vi "Open.vi"(8 "error in (no error)":errorcluster caption="entrée d'erreur (pas d'erreur)", 11 "Class Power_Supply Rigol DP800 en entrée":refnum<class "Class Power_Supply Rigol DP800.lvclass">) -> (0 "error out":errorcluster caption="sortie d'erreur", 3 "Class Power_Supply Rigol DP800 en sortie":refnum<class "Class Power_Supply Rigol DP800.lvclass">)   [LabVIEW 2020, in "Library Instrument & Equipement.lvlib" / "Library Power_Supply.lvlib" / "Class Power_Supply Rigol DP800.lvclass"]
uses:
  Class Power_Supply Rigol DP800.lvclass
  C:/Users/ngarcin/OneDrive - Altyor/Standard TB/Class/Power_Supply/Power_Supply (Default)/Power_Supply (Default).lvclass
  Commun VI/TypeDef/Liste Error.ctl
  Class Power_Supply Rigol DP800.lvclass/Class Power_Supply Rigol DP800.ctl
  RIGOL DP800 Series/RIGOL DP800 Series.lvlib
  Commun VI/Library Commun.lvlib
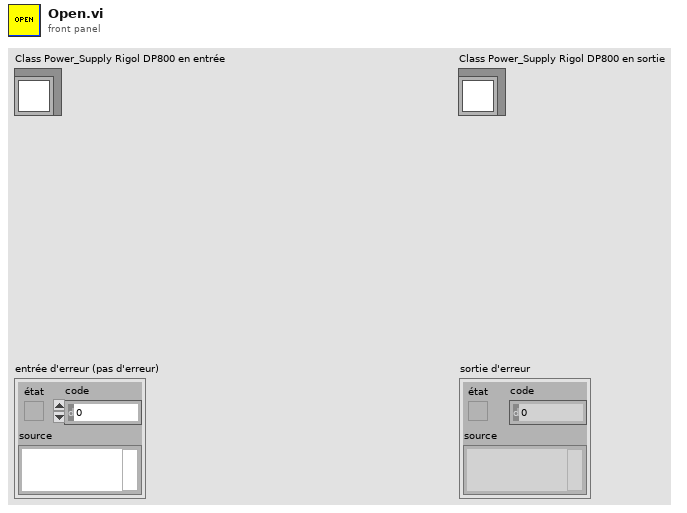
[diagram p1: front panel]
types:
  T1 = typedef "Library Commun.lvlib/Liste Error.ctl" = enum16{"Firebase Driver - Get Document", "Firebase Driver - Get Document With Where", "Firebase Driver - Delete Document", "Firebase Driver - Set Document", "Firebase Driver - Update Document", "Firebase Altyor - Search Document Bench", "Firebase Altyor - Class Not in Firebase", "Spectrum_Analyser - Timeout", "Relay Board - Qty Relay", "DIO - Pb Funtion", "Power_Supply - Peripherical not find", "Mutimeter - Peripherical not find", "Instrument - Function Not Used", "Instrument - Instrument name not specified", "Instrument - Allready Initialised", "Instrument - TimeOut", "Instrument - the instrument must be Initialise before", "Instrument - Frame Not received", "Instrument - Frame Nok", "Test - Initialise the File_for_Save", "Test - Timeout", "Test - Cmd Error", "FGV - Variable ", "BDD FireBase - Define Class", "SN - Class Not Define"}
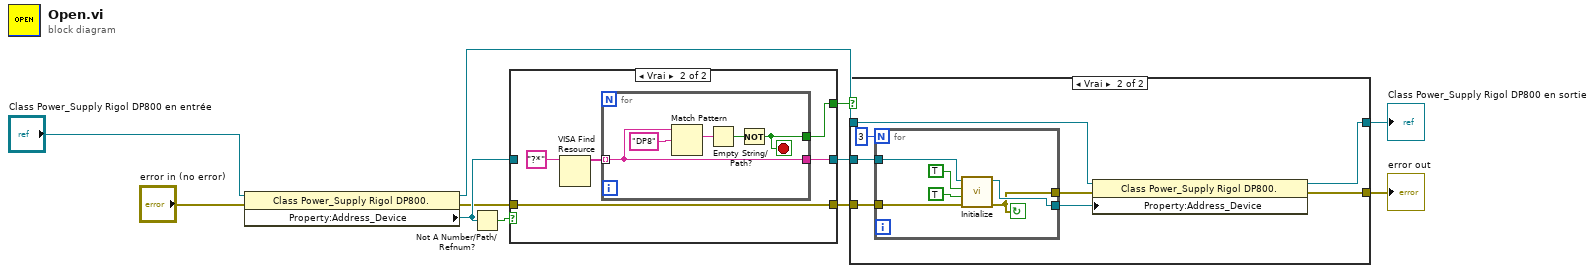
[diagram p0: block diagram]
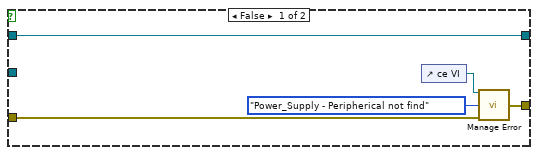
[diagram p2: hidden frame]
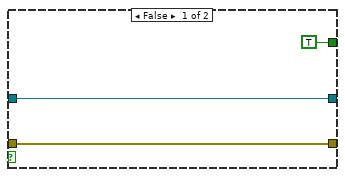
[diagram p3: hidden frame]
diagram:
  n1 = property class="Class Power_Supply Rigol DP800."(reference="Class Power_Supply Rigol DP800 en entrée", error in="error in (no error)") -> (reference out=w3:refnum<class "Class Power_Supply Rigol DP800.lvclass">, error out=w5:errorcluster, "Property:Address_Device"=w7:refnum<visa-resource-name>)
  n2 = Not A Number/Path/Refnum?(number/path/refnum=w7) -> (NaN/Path/Refnum?=w9:bool)
  n3 = case shown="Vrai" w9 {
    tunnel: [TRUE w17] -> w8
    tunnel: [w13 w16] -> w6
    tunnel: w7 -> [w13 _]
    tunnel: w5 -> [w12 w15]
    tunnel: [w12 w15] -> w4
    frame False {
    }
    frame True {
      n4 = VISA Find Resource(11:"?*" ("expression  (\"?*\")")) -> (3:w18:string[])  [unwired: 2 in, 2 out]
      n5 = for {
        tunnel: w18 -> [w21] mode=indexing
        tunnel: [w21] -> w16
        tunnel: [w20] -> w17
        stop <- w20 stop-if-true
        n6 = Match Pattern(string=w21, regular expression="DP8" ("expression régulière")) -> (match substring=w23:string)  [unwired: 1 in, 3 out]
        n7 = Empty String/Path?(string/path=w23) -> (empty?=w22:bool)
        n8 = Not(x=w22) -> (.not. x?=w20:bool)
      }
    }
  }
  n9 = case shown="Vrai" w8 {
    tunnel: w4 -> [w25 w37]
    tunnel: w6 -> [_ w33]
    tunnel: w3 -> [w26 w36]
    tunnel: [w26 w35] -> w2
    tunnel: [w27 w34] -> w1
    frame False {
      n10 = control-ref of="ce VI"() -> (w29:refnum<vi>)
      n11 = call "Manage Error.vi"("VI in Error"=w29, "Code Erreur"=Liste_Error."Power_Supply - Peripherical not find", "error in (no error)"=w25) -> ("error out"=w27:errorcluster)  [unwired: 12 in]
    }
    frame True {
      n12 = for {
        N: 3 -> [_]
        tunnel: w37 -> [w43]
        tunnel: [w38] -> w32
        tunnel: w33 -> [w42]
        tunnel: [w41] -> w31
        stop <- w38 continue-if-true
        n13 = call "Initialize.vi"("error in (no error)"=w43, "Reset (True)"=TRUE, "ID Query (True)"=TRUE, "VISA resource name"=w42) -> ("error out"=w38:errorcluster, "VISA resource name out"=w41:refnum<visa-resource-name>)  [unwired: 6 in]
      }
      n14 = property class="Class Power_Supply Rigol DP800."(reference=w36, error in=w32, "Property:Address_Device"=w31) -> (reference out=w35:refnum<class "Class Power_Supply Rigol DP800.lvclass">, error out=w34:errorcluster)
    }
  }
  "error out" <- w1
  "Class Power_Supply Rigol DP800 en sortie" <- w2
